vi "Expected Binary Version.vi"() -> (0 "Expected Version":string="1.4")   [LabVIEW 2020, in "common.lvlib"]
uses:
  common.lvlib
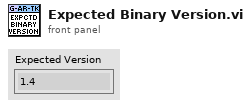
[diagram p1: front panel]
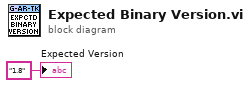
[diagram p0: block diagram]
diagram:
  "Expected Version" <- "1.8"
